vi "TargetCapture.vi"(0 "DO Task":refnum<k21>="BlueSimple_DO_All", 1 "Touch lines":T2={"Home touch"=0, "Touch 1"=1, "Touch 2"=2, "Touch 3"=3, "Touch 4"=4}, 2 "DI Task":refnum<k21>, 5 "Home+target OK?":bool, 7 "Response time":cluster{"Fix":dbl, "Rnd":dbl}={"Fix"=1.5, "Rnd"=0.0} {"Rnd" format="%.4f"; "Fix" format="%.4f"}, 9 "Tone duration":cluster{"Fix":dbl, "Rnd":dbl}={"Fix"=0.5, "Rnd"=0.0} {"Rnd" format="%.4f"; "Fix" format="%.4f"}, 11 "LED C duration":cluster{"Fix":dbl, "Rnd":dbl}={"Fix"=0.5, "Rnd"=0.0} caption="LED duration" {"Rnd" format="%.4f"; "Fix" format="%.4f"}, 12 "Target":i16, 13 "Cue brightness":i16=6 caption="Brightness", 14 "Initialize?":bool) -> (4 "Go to stage":T1(ring), 15 "Last trial successful?":bool)   [LabVIEW 2010]
uses:
  Controls/Bits to Write.ctl
panel:
  # "+"
  # "+"
  # "+"
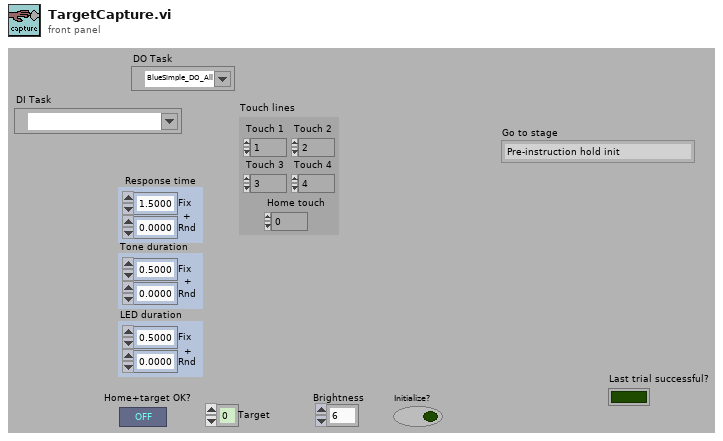
[diagram p1: front panel]
types:
  T1 = enum16{"Pre-instruction hold init", "Pre-instruction hold", "Instruction init", "Instruction", "Post-instruction hold init", "Post-instruction hold", "Target capture init", "Target capture", "Target hold init", "Target hold", "Reward stage", "Intertrial"}
  T2 = cluster{"Home touch":i16, "Touch 1":i16, "Touch 2":i16, "Touch 3":i16, "Touch 4":i16}
  T3 = typedef "Bits to Write.ctl" = enum16{"LED 1 on", "LED 1 off", "LED 2 on", "LED 2 off", "LED 3 on", "LED 3 off", "LED 4 on", "LED 4 off", "All LEDs on", "All LEDs off", "In trial on", "In trial off", "Buzzer on", "Buzzer off", "Reward on", "Reward off", "Target number", "Trial type preQ on", "Trial type preQ off", "Error on", "Error off", "Trial number", "DBS on", "DBS off", "Sine on", "Sine off", "All Bits On", "All Bits Off", "Init", "Specify mask/pattern"}
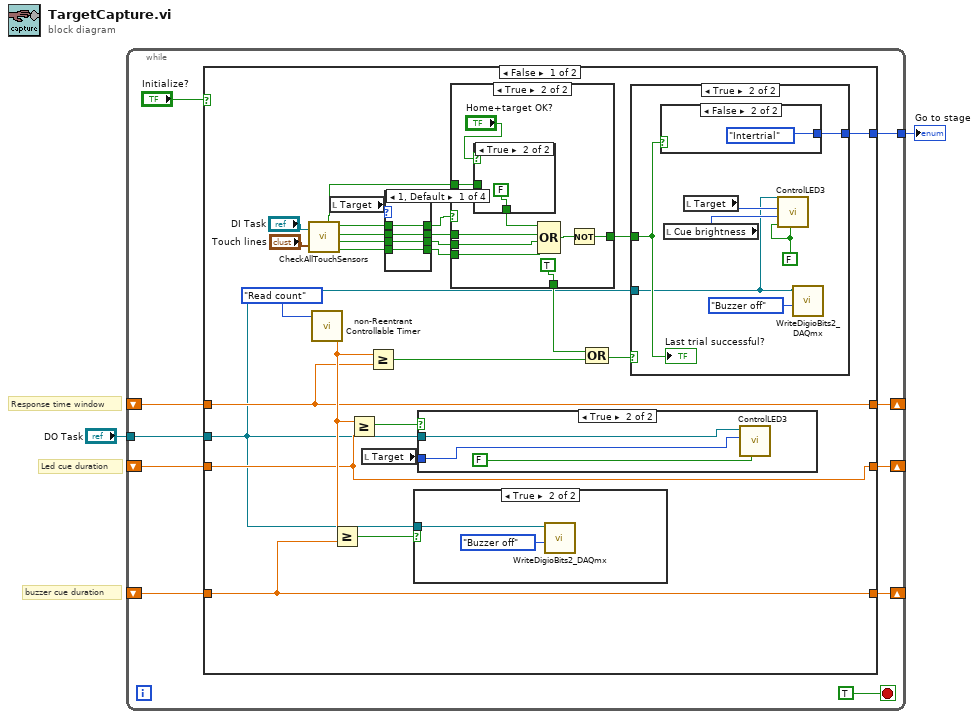
[diagram p0: block diagram]
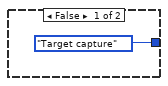
[diagram p2: hidden frame]
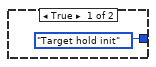
[diagram p3: hidden frame]
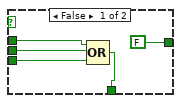
[diagram p5: hidden frame]
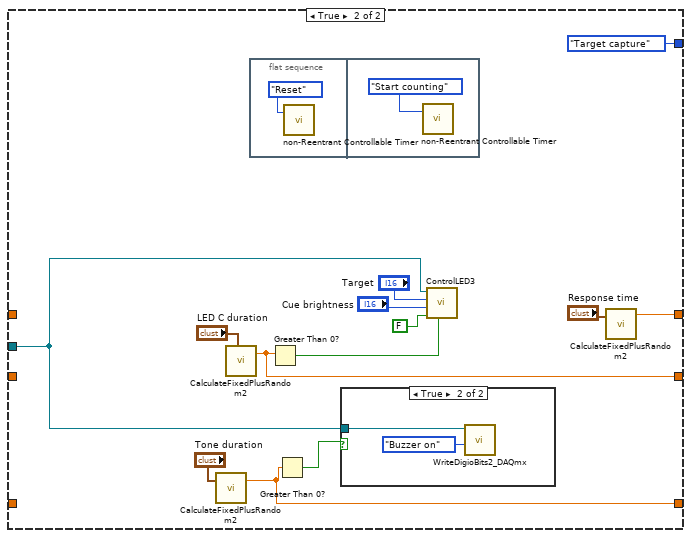
[diagram p11: hidden frame]
diagram:
  # "buzzer cue duration"
  # "Led cue duration"
  # "Response time window"
  n1 = while {
    shift-right: [w10] -> _
    shift-left: _ -> [w7]
    shift-right: [w9] -> _
    shift-left: _ -> [w6]
    shift-right: [w8] -> _
    shift-left: _ -> [w5]
    tunnel: [w4] -> w2
    tunnel: "DO Task" -> [w3]
    stop <- TRUE stop-if-true
    n2 = case shown="False" "Initialize?" {
      tunnel: [w19 w95] -> w10
      tunnel: [w18 w94] -> w9
      tunnel: [w17 w93] -> w8
      tunnel: w7 -> [w19 _]
      tunnel: w6 -> [w18 _]
      tunnel: w5 -> [w17 _]
      tunnel: [w15 T1."Target capture" ("Current stage")] -> w4
      tunnel: w3 -> [w14 w86]
      frame False {
        n3 = call "CheckAllTouchSensors.vi"("Touch sensor lines"="Touch lines", "DI Task"="DI Task") -> ("TS 4"=w31:bool, "TS 3"=w32:bool, "TS 2"=w33:bool, "TS 1"=w34:bool, "Home?"=w29:bool)
        n4 = call "non-Reentrant Controllable Timer.vi"("Enum"=enum16{"Start counting", "Read count", "Reset"}."Read count") -> ("Time out"=w24:dbl)  [unwired: 1 in]
        n5 = local read "Target"() -> (w35:i16)
        n6 = Greater Or Equal?(x=w24, y=w17) -> (x >= y?=w20:bool)
        n7 = Greater Or Equal?(x=w24, y=w18) -> (x >= y?=w21:bool)
        n8 = local read "Target"() -> (w37:i16)
        n9 = Greater Or Equal?(x=w24, y=w19) -> (x >= y?=w36:bool)
        n10 = case shown="1, Default" w35 {
          tunnel: w34 -> [w71 w74 w78 w82]
          tunnel: w33 -> [w70 w75 w77 w81]
          tunnel: w32 -> [w69 w73 w79 w80]
          tunnel: w31 -> [w68 w72 w76 w83]
          tunnel: [w71 w75 w79 w83] -> w30
          tunnel: [w70 w74 w78 w82] -> w28
          tunnel: [w69 w73 w77 w81] -> w27
          tunnel: [w68 w72 w76 w80] -> w26
          frame 1, Default {
          }
          frame 2 {
          }
          frame 3 {
          }
          frame 4 {
          }
        }
        n11 = case shown="True" w20 {
          tunnel: w14 -> [_ w84]
          frame False {
          }
          frame True {
            n12 = call "WriteDigioBits2_DAQmx.vi"("Bits to write"=Bits_to_Write."Buzzer off", "DO Task"=w84) -> ()  [unwired: 9 in, 1 out]
          }
        }
        n13 = case shown="True" w21 {
          tunnel: w37 -> [_ w50]
          tunnel: w14 -> [_ w49]
          frame False {
          }
          frame True {
            n14 = call "ControlLED3.vi"("On?"=FALSE ("Line state"), "Target"=w50, "DO Task"=w49) -> ()  [unwired: 8 in]
          }
        }
        n15 = case shown="True" w30 {
          tunnel: w29 -> [_ w58]
          tunnel: w28 -> [w54 w65]
          tunnel: w27 -> [w55 w64]
          tunnel: w26 -> [w56 w63]
          tunnel: [w53 TRUE] -> w25
          tunnel: [FALSE w61] -> w38
          frame False {
            n16 = Compound Arithmetic op=OR(w54, w55, w56) -> (w53:bool)
          }
          frame True {
            n17 = case shown="True" "Home+target OK?" {
              tunnel: [w66 FALSE ("Home?")] -> w57
              tunnel: w58 -> [w66 _]
              frame False {
              }
              frame True {
              }
            }
            n18 = Compound Arithmetic op=OR(w57, w65, w64, w63) -> (w62:bool)
            n19 = Not(x=w62) -> (.not. x?=w61:bool)
          }
        }
        n20 = Compound Arithmetic op=OR(w25, w36) -> (w16:bool)
        n21 = case shown="True" w16 {
          tunnel: w38 -> [_ w46]
          tunnel: [T1."Target capture" ("Current stage") w45] -> w15
          tunnel: w14 -> [_ w40]
          frame False {
          }
          frame True {
            w42 = FALSE ("Line state")
            n22 = case shown="False" w46 {
              tunnel: [T1."Target hold init" ("Current stage") T1."Intertrial" ("Current stage")] -> w45
              frame True {
              }
              frame False {
              }
            }
            n23 = local read "Cue brightness"() -> (w43:i16)
            n24 = local read "Target"() -> (w44:i16)
            n25 = call "ControlLED3.vi"("On?"=w42, "All flash?"=w42, "Brightness"=w43, "Target"=w44, "DO Task"=w40) -> ()  [unwired: 6 in]
            n26 = call "WriteDigioBits2_DAQmx.vi"("Bits to write"=Bits_to_Write."Buzzer off", "DO Task"=w40) -> ()  [unwired: 9 in, 1 out]
            "Last trial successful?" <- w46
          }
        }
      }
      frame True {
        n27 = call "CalculateFixedPlusRandom2.vi"("Component times"="Tone duration") -> ("Composite time"=w93:dbl)  [unwired: 1 in, 1 out]
        n28 = call "CalculateFixedPlusRandom2.vi"("Component times"="LED C duration") -> ("Composite time"=w94:dbl)  [unwired: 1 in, 1 out]
        n29 = flat-sequence {
          frame #0 {
            n30 = call "non-Reentrant Controllable Timer.vi"("Enum"=enum16{"Start counting", "Read count", "Reset"}."Reset") -> ()  [unwired: 1 in, 1 out]
          }
          frame #1 {
            n31 = call "non-Reentrant Controllable Timer.vi"("Enum"=enum16{"Start counting", "Read count", "Reset"}."Start counting") -> ()  [unwired: 1 in, 1 out]
          }
        }
        n32 = Greater Than 0?(x=w94) -> (x > 0?=w89:bool)
        n33 = Greater Than 0?(x=w93) -> (x > 0?=w87:bool)
        n34 = case shown="True" w87 {
          tunnel: w86 -> [_ w99]
          frame False {
          }
          frame True {
            n35 = call "WriteDigioBits2_DAQmx.vi"("Bits to write"=Bits_to_Write."Buzzer on", "DO Task"=w99) -> ()  [unwired: 9 in, 1 out]
          }
        }
        n36 = call "ControlLED3.vi"("On?"=w89, "All flash?"=FALSE, "Brightness"="Cue brightness", "Target"="Target", "DO Task"=w86) -> ()  [unwired: 6 in]
        n37 = call "CalculateFixedPlusRandom2.vi"("Component times"="Response time") -> ("Composite time"=w95:dbl)  [unwired: 1 in, 1 out]
      }
    }
  }
  "Go to stage" <- w2
